vi "sendcommand.vi"(6 "addr/port":cluster{"address":string, "port":i32}, 8 "error in (no error)":errorcluster, 11 "command":string) -> (0 "error out":errorcluster, 2 "bytes written":i32, 3 "connection ID out":refnum<k5>)   [LabVIEW 2015]
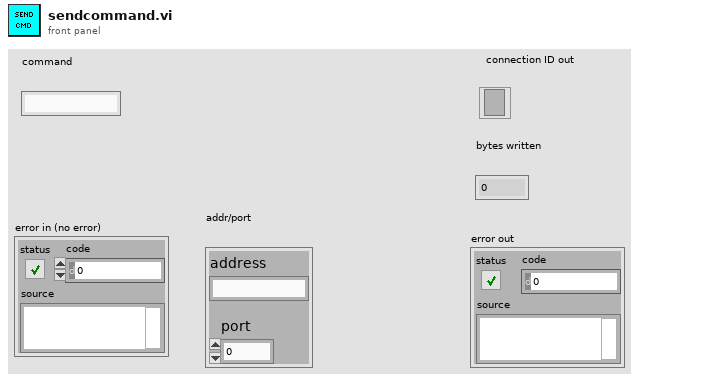
[diagram p1: front panel]
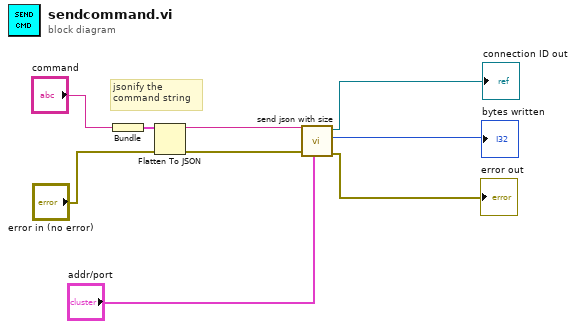
[diagram p0: block diagram]
diagram:
  # "jsonify the \ncommand string"
  n1 = Bundle("command"="command") -> (w7:cluster{"command":string})  [unwired: 1 in]
  n2 = Flatten To JSON(anything=w7, error in (no error)="error in (no error)") -> (JSON string=w5:string, 11:w6:errorcluster)  [unwired: 1 in]
  n3 = call "send json with size.vi"("addr/port"="addr/port", "error in"=w6, "json string"=w5) -> ("error out"=→"error out":errorcluster, "bytes written"=→"bytes written":i32, "connection ID out"=→"connection ID out":refnum<k5>)  [unwired: 6 in]
